vi "Calc_Roller.vi"(10 "Roller Commands":T1, 11 "Accepting Balls?":bool) -> (3 "Roller Outputs":T2)   [LabVIEW 2012]
uses:
  Outputs_Roller.ctl
  Input_Commands_Roller.ctl
panel:
  in  "Roller Speed":dbl=0.35
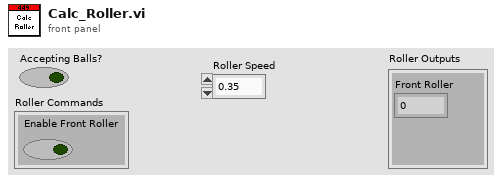
[diagram p1: front panel]
types:
  T1 = typedef "Input_Commands_Roller.ctl" = cluster{"Enable Front Roller":bool}
  T2 = typedef "Outputs_Roller.ctl" = cluster{"Front Roller":dbl}
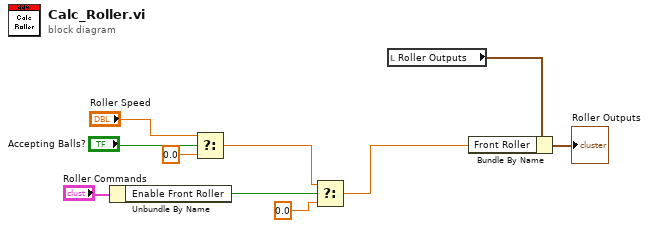
[diagram p0: block diagram]
diagram:
  n1 = Unbundle By Name("Roller Commands") -> ("Enable Front Roller"=w6:bool)
  n2 = Select(t="Roller Speed", s="Accepting Balls?", f=0.0) -> (s? t:f=w3:dbl)
  n3 = Select(t=w3, s=w6, f=0.0) -> (s? t:f=w2:dbl)
  n4 = local read "Roller Outputs"() -> (w9:T2)
  n5 = Bundle By Name(cluster=w9, "Front Roller"=w2) -> (→"Roller Outputs":T2)
